vi "Report Event.vi"(7 "Level (Info)":T1=enum."Info", 8 "error in (no error)":errorcluster, 9 "Message":string, 11 "Module in":refnum<class "Module.lvclass">) -> (0 "error out":errorcluster, 3 "Module out":refnum<class "Module.lvclass">)   [LabVIEW 2020, in "Volatus.lvlib" / "Module.lvclass"]
uses:
  Module.lvclass
  Event Level.ctl
  Module.lvclass/Module.ctl
  VolatusAPI/VolatusAPI.lvclass
  Volatus.lvlib
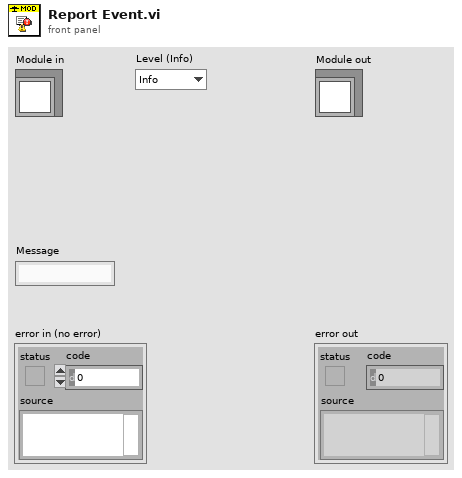
[diagram p1: front panel]
types:
  T1 = typedef "Volatus.lvlib/Event Level.ctl" = enum16{"Debug", "Info", "Warning", "Error"}
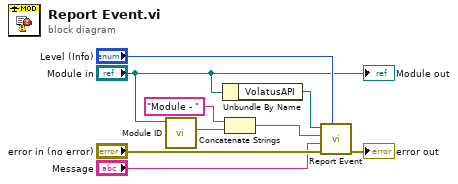
[diagram p0: block diagram]
diagram:
  n1 = call-dynamic "Module ID.vi"("Module in"="Module in") -> ("Module ID"=w4:string)  [unwired: 10 in]
  n2 = Unbundle By Name("Module in") -> ("VolatusAPI"=w9:refnum<class "VolatusAPI.lvclass">)
  n3 = Concatenate Strings("Module - ", w4) -> (w2:string)
  n4 = call "Report Event.vi"("Level (Info)"="Level (Info)", "error in (no error)"="error in (no error)", "Message"="Message", "Context"=w2, "VolatusAPI in"=w9) -> ("error out"=→"error out":errorcluster)  [unwired: 5 in, 1 out]
  "Module out" <- "Module in"
